vi "WriteHeader.vi"(8 "error in (no error)":errorcluster, 11 "SimpleErrorLogger in":refnum<class "SimpleErrorLogger.lvclass">) -> (0 "error out":errorcluster, 3 "SimpleErrorLogger out":refnum<class "SimpleErrorLogger.lvclass">)   [LabVIEW 2023, in "SimpleErrorLogger.lvlib" / "SimpleErrorLogger.lvclass"]
uses:
  SimpleErrorLogger.lvclass
  SimpleErrorLogger.lvclass/SimpleErrorLogger.ctl
  <vilib>/ActorFramework/Actor/Actor.lvclass/Actor.ctl
  <vilib>/ActorFramework/Message Enqueuer/Message Enqueuer.lvclass/Message Enqueuer.ctl
  <vilib>/ActorFramework/Message Enqueuer/Init from Existing Queue.vi
  <vilib>/ActorFramework/Message Enqueuer/Enqueue.vi
  SimpleErrorLogger Messages/Open Msg/Open Msg.lvclass
  <vilib>/ActorFramework/Message Priority Queue/Priority Enqueue.vi
  <vilib>/ActorFramework/Message Enqueuer/Message Enqueuer.lvclass
  <vilib>/ActorFramework/Actor/Actor.lvclass
  C:/Program Files (x86)/National Instruments/LabVIEW 2023/vi.lib/ActorFramework/Actor/Actor.lvclass
  C:/Source/LabVIEW/Error_Logger/SimpleErrorLogger/SimpleErrorLogger/SimpleErrorLogger.lvclass
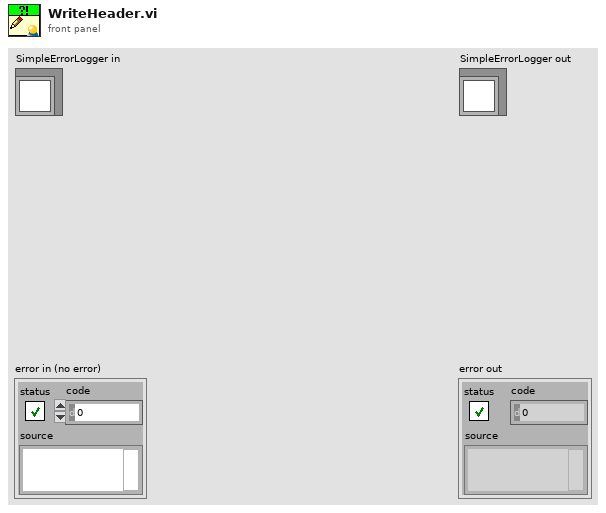
[diagram p1: front panel]
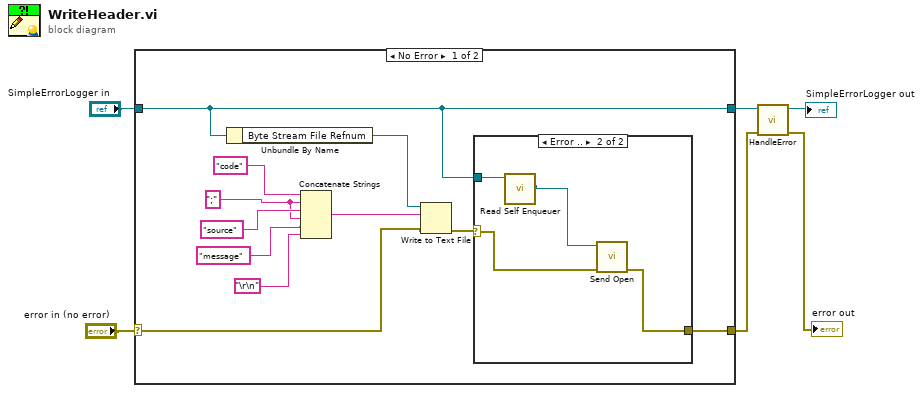
[diagram p0: block diagram]
diagram:
  n1 = case shown="No Error" "error in (no error)" {
    selector: "error in (no error)" -> [w10 w24]
    tunnel: [w8 w24] -> w2
    tunnel: [w7 w23] -> w4
    tunnel: "SimpleErrorLogger in" -> [w7 w23]
    frame No Error {
      w14 = ";" ("string")
      n2 = Unbundle By Name(w7) -> ("Byte Stream File Refnum"=w17:refnum<file>)
      n3 = Concatenate Strings("code" ("string"), w14, "source" ("string"), w14, "message" ("string"), "\r\n") -> (w11:string)
      n4 = Write to Text File(file (use dialog)=w17, text=w11, error in=w10) -> (error out=w9:errorcluster)  [unwired: 1 in, 2 out]
      n5 = case shown="Error .." w9 {
        selector: w9 -> [w18 w20]
        tunnel: [w18 w19] -> w8
        tunnel: w7 -> [_ w22]
        frame No Error {
        }
        frame Error {
          n6 = call <vilib>:"Read Self Enqueuer.vi"("Actor"=w22) -> ("Self Enqueuer"=w21:refnum<class "Message Enqueuer.lvclass">)  [unwired: 10 in]
          n7 = call "Send Open.vi"("error in (no error)"=w20, "Message Enqueuer"=w21) -> ("error out"=w19:errorcluster)  [unwired: 8 in, 1 out]
        }
      }
    }
    frame Error {
    }
  }
  n8 = call "HandleError.vi"("error in (no error)"=w2, "SimpleErrorLogger in"=w4) -> ("error out"=→"error out":errorcluster, "SimpleErrorLogger out"=→"SimpleErrorLogger out":refnum<class "SimpleErrorLogger.lvclass">)  [unwired: 8 in]
